vi "Set Enable State on Multiple Controls.vi"(0 "Control References":refnum<vi>[](array[refnum]), 5 "State":T1(ring), 11 "error in":errorcluster) -> (4 "Control References dup":refnum<vi>[](array[refnum]), 15 "error out":errorcluster)   [LabVIEW 2017, in "CL_G3_BuilderApplicationLayer.lvlib"]
uses:
  CL_G3_BuilderApplicationLayer.lvlib
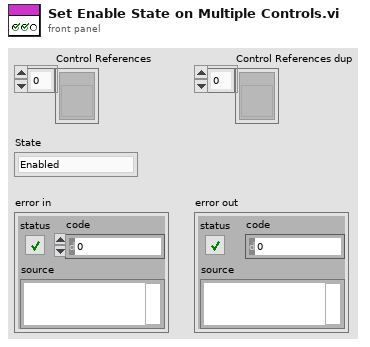
[diagram p1: front panel]
types:
  T1 = enum8{"Enabled", "Disabled", "Disabled and Grayed Out"}
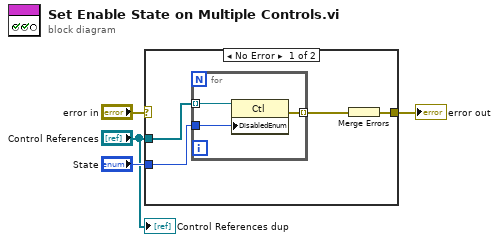
[diagram p0: block diagram]
diagram:
  n1 = case shown="No Error" "error in" {
    selector: "error in" -> [_ w12]
    tunnel: "State" -> [w8 _]
    tunnel: "Control References" -> [w7 _]
    tunnel: [w5 w12] -> w2
    frame No Error {
      n2 = for {
        tunnel: w7 -> [w11] mode=indexing
        tunnel: w8 -> [w10]
        tunnel: [w9] -> w6 mode=indexing
        n3 = property class="Ctl"(reference=w11, "DisabledEnum"=w10) -> (error out=w9:errorcluster)  [unwired: 1 in, 1 out]
      }
      n4 = Merge Errors(w6) -> (w5:errorcluster)
    }
    frame Error {
    }
  }
  "error out" <- w2
  "Control References dup" <- "Control References"
